vi "Time.Inline Record Start Time Secs.vi"(8 "Error Out Lower":errorcluster, 11 "Error In Upper":errorcluster) -> (0 "Error Out Upper":errorcluster, 1 "Start(s)":dbl, 3 "Error Out Upper":errorcluster)   [LabVIEW 2024, in "EQMF.lvlib" / "Time Utils.lvlib"]
uses:
  Time Utils.lvlib
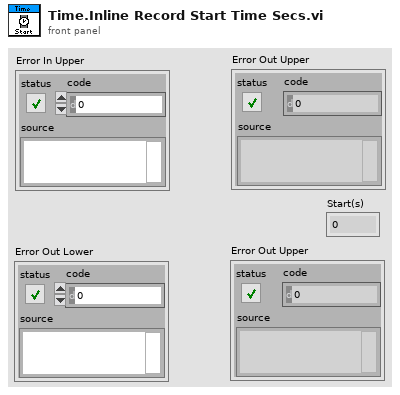
[diagram p1: front panel]
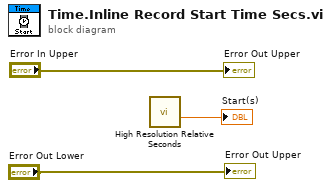
[diagram p0: block diagram]
diagram:
  n1 = call <vilib>:"High Resolution Relative Seconds.vi"() -> ("relative seconds"=→"Start(s)":dbl)
  "Error Out Upper" <- "Error In Upper"
  "Error Out Upper" <- "Error Out Lower"
